vi "Run Action_Do.vi"(8 "error in (no error)":errorcluster, 10 "Action Data":T1, 11 "Report Handler in":refnum<class "Report Handler.lvclass">) -> (0 "error out":errorcluster, 1 "Success?":bool, 3 "Report Interface out":refnum<class "Report Data.lvclass">)   [LabVIEW 2020, in "ProjectBuilder.lvlib" / "Report Handler.lvclass"]
uses:
  Report Data/Report Data.lvclass
  Ctl/Ctl_Action Data.ctl
  Report Handler.lvclass
  ProjectBuilder.lvlib
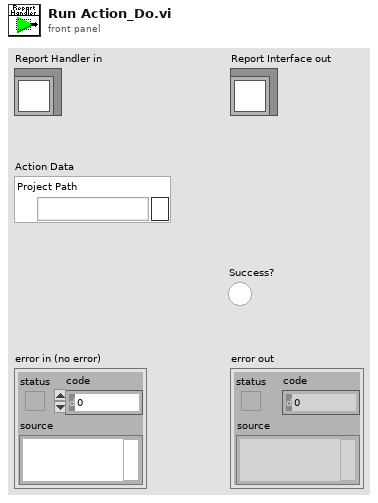
[diagram p1: front panel]
types:
  T1 = typedef "ProjectBuilder.lvlib/Ctl_Action Data.ctl" = cluster{"Project Path":path}
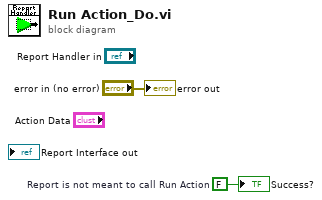
[diagram p0: block diagram]
diagram:
  w2 = FALSE  # Report is not meant to call Run Action
  "error out" <- "error in (no error)"
  "Success?" <- w2
